vi "Far to Line1.vi"(6 "Command Info In":T1, 7 "Speed":dbl, 8 "Distance":dbl, 9 "Target Angle":dbl format="%#_13g") -> (0 "Command Info Out":T1)   [LabVIEW 2017]
uses:
  <vilib>/Rock Robotics/WPI/Framework/Command Status Info.ctl
  <vilib>/Rock Robotics/WPI/Framework/Completion Status.ctl
  <vilib>/Rock Robotics/WPI/Framework/Completion Notifier.ctl
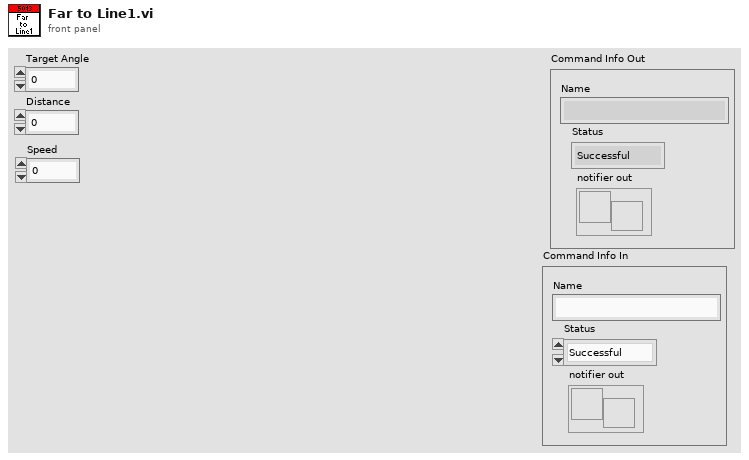
[diagram p1: front panel]
types:
  T1 = typedef "Command Status Info.ctl" = cluster{"Name":string, "Status":T2, "notifier out":T3}
  T2 = typedef "Completion Status.ctl" = enum16{"Successful", "Aborted", "Incomplete"}
  T3 = typedef "Completion Notifier.ctl" = refnum<notifier>
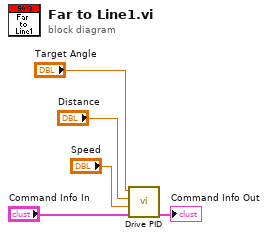
[diagram p0: block diagram]
diagram:
  n1 = call "Drive PID.vi"("Command Info In"="Command Info In", "Speed"="Speed", "Distance"="Distance", "Target Angle"="Target Angle") -> ("Command Info Out"=→"Command Info Out":T1)  [unwired: 7 in]
